vi "Pack4_UNDT.vi"(8 "ClusterIn":T3={"Header size"=56, "MagicWord"=305419896, "byte order"=enum."little-endian", "Проверка конца пакета"=TRUE, "Проверка CRC8"=TRUE, "LastPacketIn"=6858, "MinimalString"=10000} {"MagicWord" format="%.0x"}, 11 "StringIn":string) -> (0 "ClusterOut":T2, 2 "Array":T1[](array[typedef]) {"Gain Coeff" format="%#_6e"; "Reserve 1" format="%02x"; "Mux TX" format="%02x"; "Mux RX" format="%02x"; "ScanDelay" format="%02x"; "PacketCounter" format="%08x"; "SamplingInterval" format="%#_6e"; "Lose Packet" format="%08x"; "EncodersParam2" format="%016x"; "EncodersParam1" format="%016x"; "CRC 8" format="%02x"; "N chanel" format="%02x"; "N tick" format="%02x"; "Ncycle" format="%04x"; "FrameFormatVersion" format="%02x"; "MagicWord" format="%.0x"}, 3 "StringLast":string)   [LabVIEW 2017]
uses:
  Control_EU/UNDT_ClusterPack (Type).ctl
panel:
  out "String":string
  out "match + rest of string":string
  out "CheckEndPack":bool
  out "PackRecived":bool
  out "PackSize":u32
  out "CheckCRC8":bool
  out "Header size":u32
  out "MWnotFund":bool
  out "MinStr":bool
  out "MinimalString":i32
  out "ErrorSizeCount":i32
  out "ErrorCRC8Count":i32
  out "ErrorCRC8":bool
  out "DataSize":u16
  out "RemainingBytes":u32
  out "OffsetMagicWord":i32
  out "DataSizeSmall":bool
  out "ErrorEndPack":bool
  out "ErrorSeqPackCount":i32
  out "ErrorSequence":bool
  out "LastPacket":u32
  out "PackGoodParsing":i32
  out "Iteration":i32
  out "MagicWordStr":string
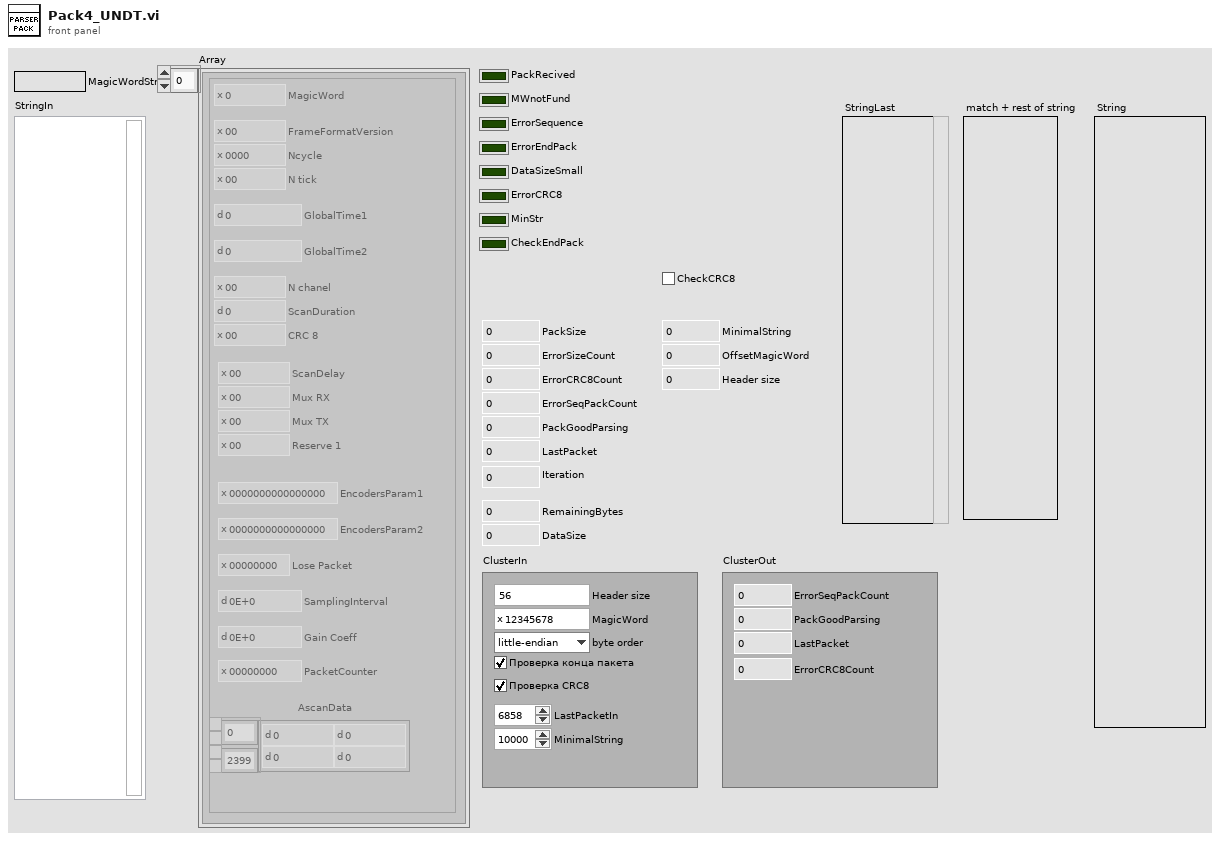
[diagram p1: front panel]
types:
  T1 = typedef "UNDT_ClusterPack (Type).ctl" = cluster{"MagicWord":u32, "FrameFormatVersion":u8, "Ncycle":u16, "N tick":u8, "GlobalTime1":u32, "GlobalTime2":u32, "N chanel":u8, "ScanDuration":u16, "CRC 8":u8, "EncodersParam1":u64, "EncodersParam2":u64, "Lose Packet":u32, "SamplingInterval":sgl, "PacketCounter":u32, "AscanData":dbl[][], "ScanDelay":u16, "Mux RX":u8, "Mux TX":u8, "Reserve 1":u8, "Gain Coeff":sgl}
  T2 = cluster{"PackGoodParsing":u32, "LastPacket":u32, "ErrorSeqPackCount":u32, "ErrorCRC8Count":u32}
  T3 = cluster{"Header size":u32, "MagicWord":u32, "byte order":enum16{"big-endian, network order", "native, host order", "little-endian"}, "Проверка конца пакета":bool, "Проверка CRC8":bool, "LastPacketIn":u32, "MinimalString":i32}
  T4 = enum16{"big-endian, network order", "native, host order", "little-endian"}
  T5 = typedef "UNDT_ClusterPackRevers (Type).ctl" = cluster{"PacketCounter":u32, "Gain Coeff":sgl, "SamplingInterval":sgl, "Lose Packet":u32, "EncodersParam2":u64, "EncodersParam1":u64, "Reserve 1":u8, "Mux TX/RX":u8, "ScanDelay":u16, "CRC 8":u8, "ScanDuration":u16, "N chanel":u8, "GlobalTime2":u32, "GlobalTime1":u32, "N tick":u8, "Ncycle":u16, "FrameFormatVersion":u8, "MagicWord":u32, "Overload":bool}
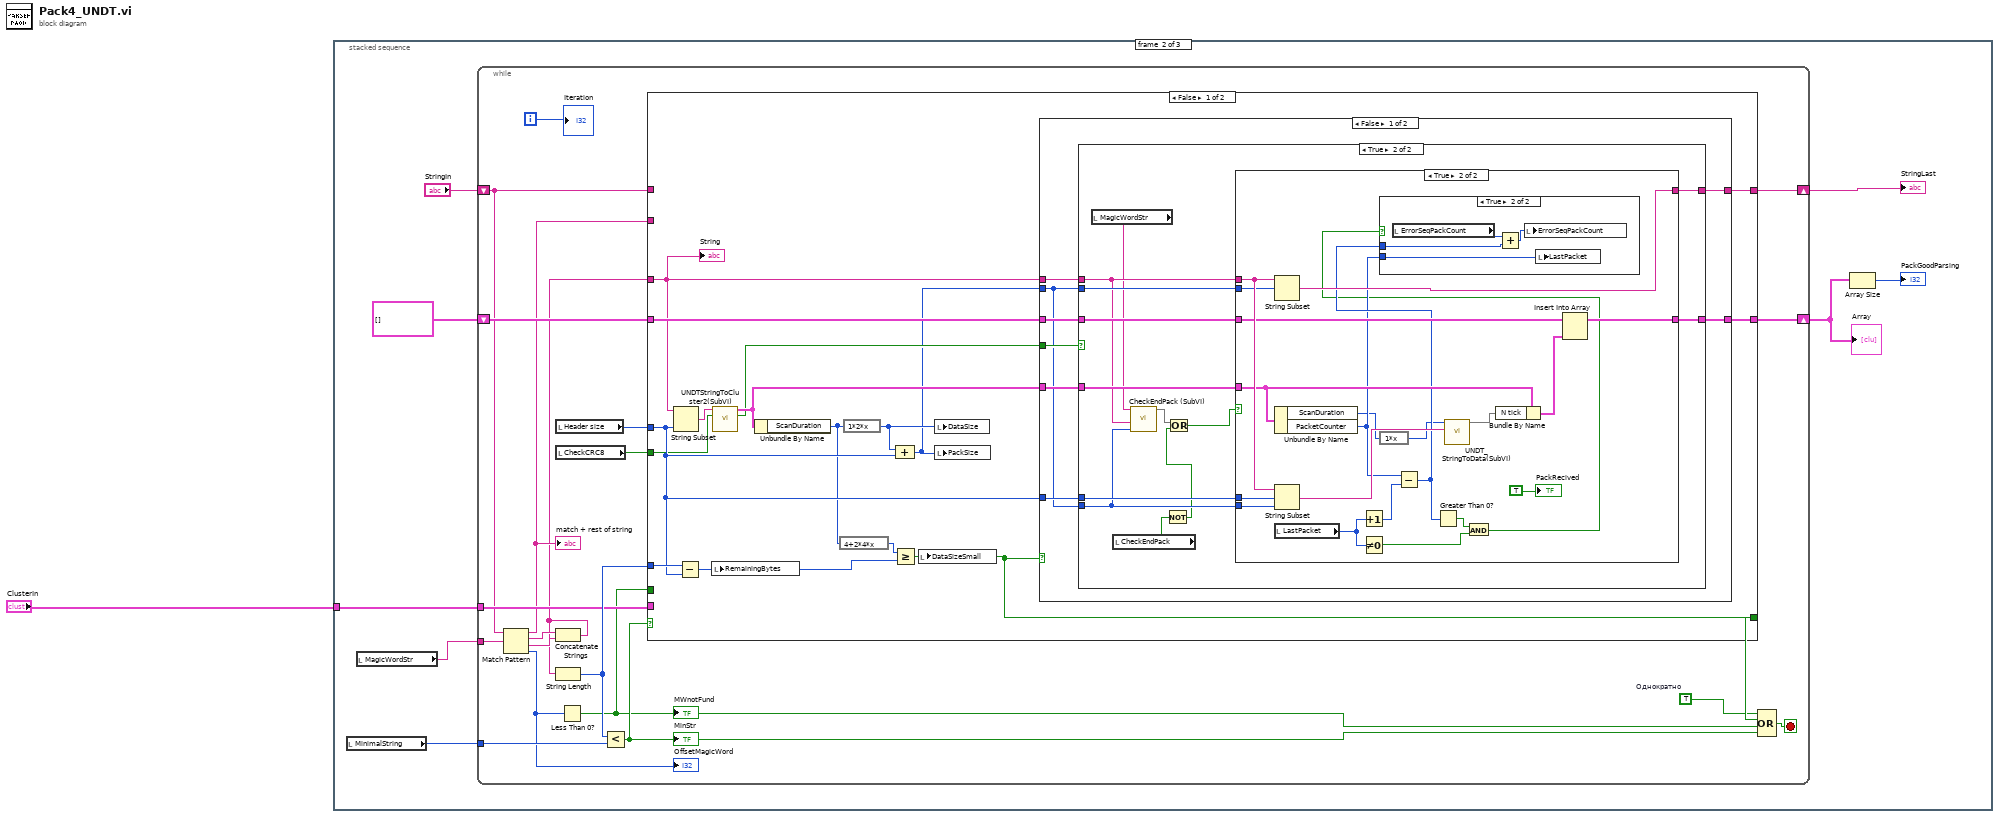
[diagram p0: block diagram]
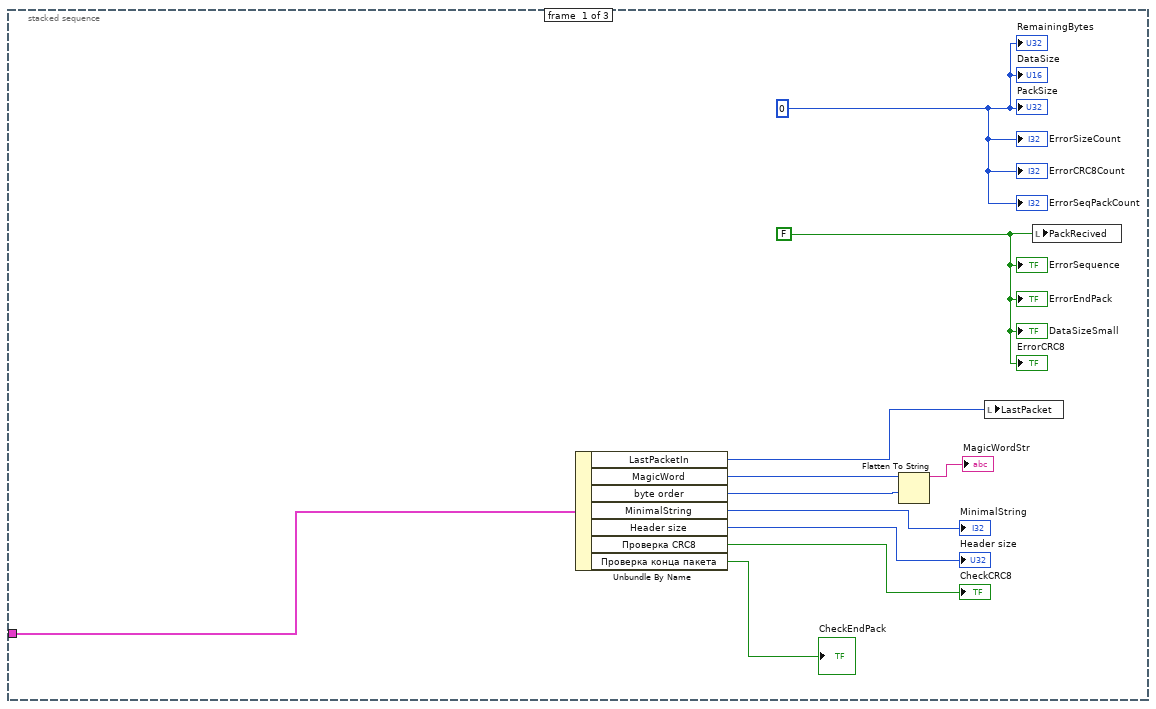
[diagram p2: hidden frame]
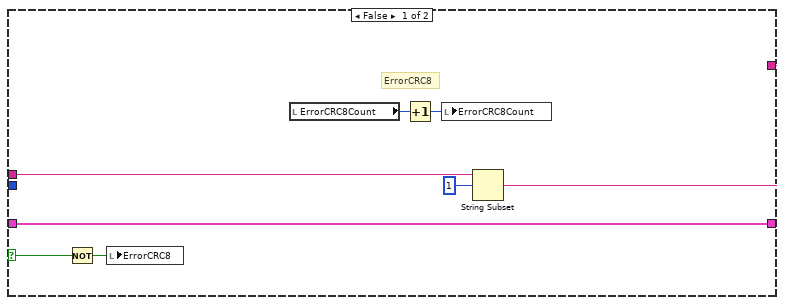
[diagram p3: hidden frame]
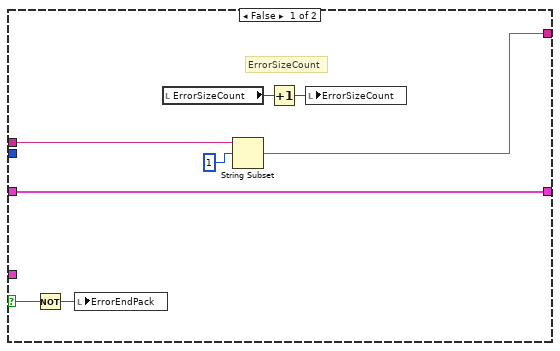
[diagram p4: hidden frame]
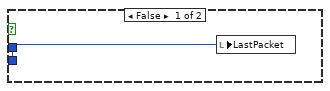
[diagram p5: hidden frame]
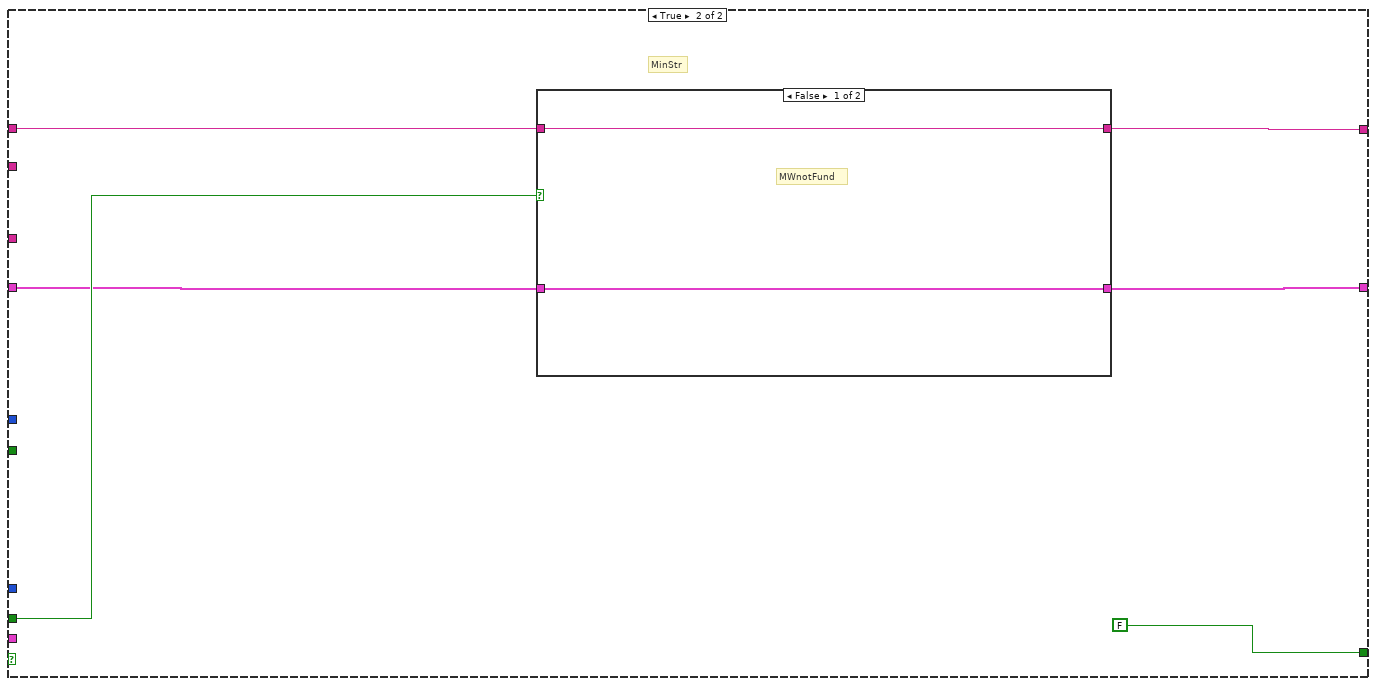
[diagram p7: hidden frame]
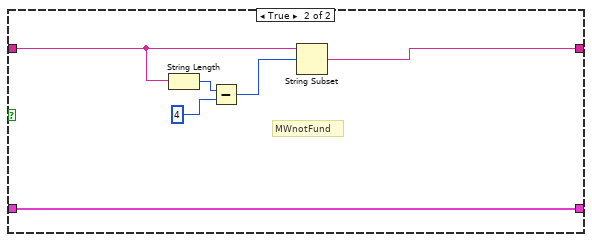
[diagram p8: hidden frame]
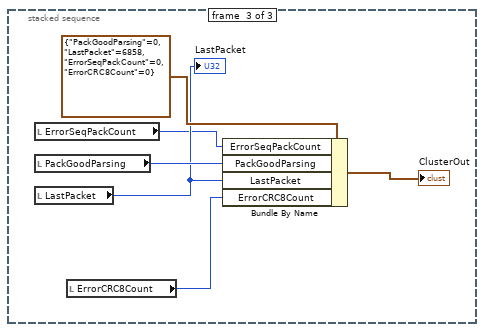
[diagram p9: hidden frame]
diagram:
  n1 = stacked-sequence {
    tunnel: "ClusterIn" -> [w3 w16 _]
    frame #0 {
      w5 = 0 ("ErrorSeqCount")
      w4 = FALSE ("PackLost")
      n2 = Unbundle By Name(w3) -> ("LastPacketIn"=w8:u32, "MagicWord"=w10:u32, "byte order"=w11:T4, "MinimalString"=→"MinimalString":i32, "Header size"=→"Header size":u32, "Проверка CRC8"=→"CheckCRC8":bool, "Проверка конца пакета"=→"CheckEndPack":bool)
      n3 = Flatten To String(anything=w10, byte order (0:big-endian, network order)=w11) -> (data string=→"MagicWordStr":string)  [unwired: 2 in, 2 out]
      n4 = local write "LastPacket"(w8) -> ()
      n5 = local write "PackRecived"(w4) -> ()
      "ErrorSequence" <- w4
      "ErrorSeqPackCount" <- w5
      "ErrorEndPack" <- w4
      "ErrorCRC8Count" <- w5
      "DataSizeSmall" <- w4
      "ErrorSizeCount" <- w5
      "RemainingBytes" <- w5
      "DataSize" <- w5
      "PackSize" <- w5
      "ErrorCRC8" <- w4
    }
    frame #1 {
      n6 = local read "MinimalString"() -> (w15:i32)
      n7 = local read "MagicWordStr"() -> (w14:string)
      n8 = while {
        tunnel: w14 -> [w25]
        shift-right: [w34] -> w20
        shift-left: "StringIn" -> [w28]
        shift-right: [w38] -> w18
        shift-left: T1[] [] -> [w37]
        tunnel: w16 -> [w36]
        tunnel: w15 -> [w35]
        i -> [w39]
        stop <- w41 stop-if-true
        w24 = TRUE  # Однократно
        n9 = Match Pattern(string=w28, regular expression=w25) -> (before substring=w27:string, match substring=w23:string, after substring=w22:string, offset past match=w26:i32)  [unwired: 1 in]
        "OffsetMagicWord" <- w26
        "match + rest of string" <- w27
        n10 = local read "Header size"() -> (w30:u32)
        n11 = local read "CheckCRC8"() -> (w29:bool)
        n12 = Concatenate Strings(w23, w22) -> (w21:string)
        n13 = String Length(string=w21) -> (length=w40:i32)
        n14 = Less Than 0?(x=w26) -> (x < 0?=w32:bool)
        "MWnotFund" <- w32
        n15 = Less?(x=w40, y=w35) -> (x < y?=w33:bool)
        "MinStr" <- w33
        n16 = case shown="False" w33 {
          tunnel: w21 -> [w48 _]
          tunnel: [w57 w125] -> w34
          tunnel: [w42 FALSE] -> w31
          tunnel: w27 -> [_ _]
          tunnel: w28 -> [_ w124]
          tunnel: w40 -> [w55 _]
          tunnel: w36 -> [_ _]
          tunnel: [w53 w127] -> w38
          tunnel: w37 -> [w52 w126]
          tunnel: w32 -> [_ w128]
          tunnel: w30 -> [w51 _]
          tunnel: w29 -> [w50 _]
          frame False {
            n17 = String Subset(string=w48, length (rest)=w51) -> (substring=w54:string)  [unwired: 1 in]
            n18 = Subtract(x=w55, y=w51) -> (x-y=w46:u32)
            n19 = local write "RemainingBytes"(w46) -> ()
            n20 = call "UNDTStringToCluster2(SubVI).vi"("Проверка CRC8"=w50, "data_in"=w54) -> ("CRC8Good"=w44:bool, "UNDT_Cluster 3"=w56:T5)  [unwired: 6 in, 2 out]
            n21 = Unbundle By Name(w56) -> ("ScanDuration"=w49:u16)
            n22 = expression code="4+2*4*x"(w49) -> (w45:u16)
            n23 = expression code="1*2*x"(w49) -> (w47:u16)
            n24 = Greater Or Equal?(x=w45, y=w46) -> (x >= y?=w42:bool)
            n25 = Compound Arithmetic op=ADD(w47, w51) -> (w43:u32)
            n26 = local write "DataSizeSmall"(w42) -> ()
            n27 = local write "DataSize"(w47) -> ()
            n28 = local write "PackSize"(w43) -> ()
            n29 = case shown="False" w42 {
              tunnel: [w65 w121] -> w57
              tunnel: w56 -> [w64 _]
              tunnel: [w63 w122] -> w53
              tunnel: w52 -> [w62 w122]
              tunnel: w51 -> [w61 _]
              tunnel: w48 -> [w60 w121]
              tunnel: w44 -> [w59 _]
              tunnel: w43 -> [w58 _]
              frame False {
                n30 = case shown="True" w59 {
                  selector: w59 -> [w66 _]
                  tunnel: [w71 w86] -> w65
                  tunnel: w64 -> [_ w85]
                  tunnel: [w72 w84] -> w63
                  tunnel: w62 -> [w72 w83]
                  tunnel: w61 -> [_ w82]
                  tunnel: w58 -> [_ w81]
                  tunnel: w60 -> [w73 w80]
                  tunnel: w58 -> [_ w79]
                  frame False {
                    # "ErrorCRC8"
                    n31 = Not(x=w66) -> (.not. x?=w67:bool)
                    n32 = local write "ErrorCRC8"(w67) -> ()
                    n33 = local read "ErrorCRC8Count"() -> (w70:i32)
                    n34 = Increment(x=w70) -> (x+1=w69:i32)
                    n35 = local write "ErrorCRC8Count"(w69) -> ()
                    n36 = String Subset(string=w73, offset (0)=1) -> (substring=w71:string)  [unwired: 1 in]
                  }
                  frame True {
                    n37 = local read "MagicWordStr"() -> (w78:string)
                    n38 = local read "CheckEndPack"() -> (w75:bool)
                    n39 = call "CheckEndPack (SubVI).vi"("error in"=w79, "OfsetEndPack"=w80, "data"=w78) -> (3:w77)  [unwired: 5 in, 3 out]
                    n40 = Not(x=w75) -> (.not. x?=w74:bool)
                    n41 = Or(x=w77, y=w74) -> (x .or. y?=w76:bool)
                    n42 = case shown="True" w76 {
                      selector: w76 -> [w87 _]
                      tunnel: [w89 w115] -> w86
                      tunnel: w80 -> [w93 w114]
                      tunnel: w85 -> [_ w113]
                      tunnel: w79 -> [_ w112]
                      tunnel: w82 -> [_ w111]
                      tunnel: w81 -> [_ w110]
                      tunnel: [w94 w109] -> w84
                      tunnel: w83 -> [w94 w108]
                      frame False {
                        # "ErrorSizeCount"
                        n43 = Not(x=w87) -> (.not. x?=w88:bool)
                        n44 = local write "ErrorEndPack"(w88) -> ()
                        n45 = local read "ErrorSizeCount"() -> (w91:i32)
                        n46 = String Subset(string=w93, offset (0)=1) -> (substring=w89:string)  [unwired: 1 in]
                        n47 = Increment(x=w91) -> (x+1=w92:i32)
                        n48 = local write "ErrorSizeCount"(w92) -> ()
                      }
                      frame True {
                        n49 = String Subset(string=w114, offset (0)=w110) -> (substring=w115:string)  [unwired: 1 in]
                        n50 = Unbundle By Name(w113) -> ("ScanDuration"=w96:u16, "PacketCounter"=w103:u32)
                        n51 = String Subset(string=w114, offset (0)=w111, length (rest)=w112) -> (substring=w107:string)
                        n52 = local read "LastPacket"() -> (w100:u32)
                        n53 = Increment(x=w100) -> (x+1=w105:u32)
                        n54 = Not Equal To 0?(x=w100) -> (x != 0?=w99:bool)
                        n55 = expression code="1*x"(w96) -> (w95:u16)
                        n56 = Subtract(x=w103, y=w105) -> (x-y=w104:u32)
                        n57 = Greater Than 0?(x=w104) -> (x > 0?=w102:bool)
                        n58 = call "UNDT_StringToData(SubVI).vi"(10:w107, "string in"=w95) -> (3:w97)  [unwired: 7 in, 2 out]
                        n59 = And(x=w102, y=w99) -> (x .and. y?=w101:bool)
                        n60 = case shown="True" w101 {
                          tunnel: w104 -> [_ w118]
                          tunnel: w103 -> [w116 w117]
                          frame False {
                            n61 = local write "LastPacket"(w116) -> ()
                          }
                          frame True {
                            n62 = local read "ErrorSeqPackCount"() -> (w120:i32)
                            n63 = Add(x=w120, y=w118) -> (x+y=w119:u32)
                            n64 = local write "ErrorSeqPackCount"(w119) -> ()
                            n65 = local write "LastPacket"(w117) -> ()
                          }
                        }
                        n66 = Bundle By Name(cluster=w113, "N tick"=w97) -> (w106:T5)
                        n67 = Insert Into Array(array=w108, new element=w106) -> (w109:T1[])  [unwired: 1 in]
                        "PackRecived" <- TRUE ("PackRecived")
                      }
                    }
                  }
                }
              }
              frame True {
              }
            }
            "String" <- w48
          }
          frame True {
            # "MinStr"
            n68 = case shown="False" w128 {
              tunnel: [w129 w136] -> w127
              tunnel: w126 -> [w129 w136]
              tunnel: [w130 w131] -> w125
              tunnel: w124 -> [w130 w135]
              frame False {
                # "MWnotFund"
              }
              frame True {
                # "MWnotFund"
                n69 = String Length(string=w135) -> (length=w134:i32)
                n70 = Subtract(x=w134, y=4) -> (x-y=w132:i32)
                n71 = String Subset(string=w135, offset (0)=w132) -> (substring=w131:string)  [unwired: 1 in]
              }
            }
          }
        }
        n72 = Compound Arithmetic op=OR(w24, w31, w32, w33) -> (w41:bool)
        "Iteration" <- w39
      }
      "StringLast" <- w20
      "Array" <- w18
      n73 = Array Size(array=w18) -> (size(s)=→"PackGoodParsing":i32)
    }
    frame #2 {
      n74 = local read "ErrorSeqPackCount"() -> (w138:i32)
      n75 = local read "PackGoodParsing"() -> (w140:i32)
      n76 = local read "LastPacket"() -> (w139:u32)
      "LastPacket" <- w139
      n77 = local read "ErrorCRC8Count"() -> (w137:i32)
      n78 = Bundle By Name(cluster=T2 {"PackGoodParsing"=0, "LastPacket"=6858, "ErrorSeqPackCount"=0, "ErrorCRC8Count"=0} ("ClusterOut"), "ErrorSeqPackCount"=w138, "PackGoodParsing"=w140, "LastPacket"=w139, "ErrorCRC8Count"=w137) -> (→"ClusterOut":T2)
    }
  }
